vi "SECoP-addPropertyDouble.vi"(8 "error in (no error)":errorcluster, 9 "property value":dbl, 10 "property name":string, 11 "DLL path (in)":T1) -> (0 "error out":errorcluster, 3 "DLL path (out)":T1)   [LabVIEW 2023, in "SECoP.lvlib"]
doc: "Call <b>\"SECoP-addPropertyDouble.vi\"</b> to append a SECoP numeric property to the last SEC node, module, command or parameter. This is a convenience function like \"SECoP-addProperty.vi\" with a numeric double.\n\n<b>DLL path</b> input and output of cluster from \"SECoP-Initialize.vi\"\n<b>property name</b> name of property\n<b>property value</b> value of the property"
uses:
  SECoP.lvlib
  SECoP-libraries.ctl
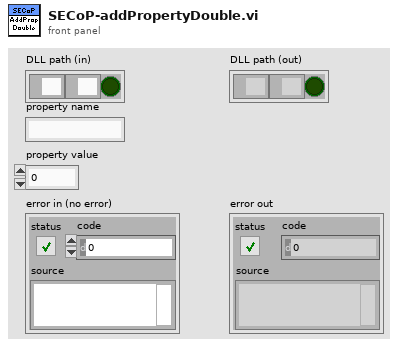
[diagram p1: front panel]
types:
  T1 = typedef "SECoP.lvlib/SECoP-libraries.ctl" = cluster{"serverDLL":path, "variantDLL":path, "cleanup_mode":bool}
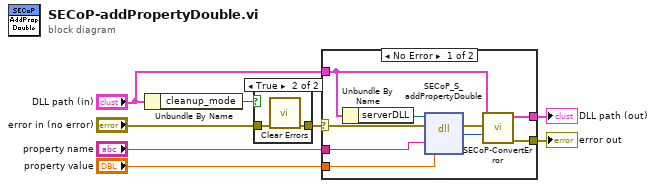
[diagram p0: block diagram]
diagram:
  n1 = Unbundle By Name("DLL path (in)") -> ("cleanup_mode"=w2:bool)
  n2 = case shown="True" w2 {
    tunnel: "error in (no error)" -> [w9 w11]
    tunnel: [w9 w10] -> w3
    frame False {
    }
    frame True {
      n3 = call <vilib>:"Clear Errors.vi"("error in (no error)"=w11) -> ("error out"=w10:errorcluster)  [unwired: 5 in, 1 out]
    }
  }
  n4 = case shown="No Error" w3 {
    selector: w3 -> [w18 w21]
    tunnel: "DLL path (in)" -> [w13 w22]
    tunnel: [w19 w22] -> w8
    tunnel: [w20 w21] -> w7
    tunnel: "property name" -> [w15 _]
    tunnel: "property value" -> [w14 _]
    frame No Error {
      n5 = Unbundle By Name(w13) -> ("serverDLL"=w12:path)
      n6 = dll-call lib="C:/Users/user/Desktop/x86_64/SECoP64.dll" fn="SECoP_S_addPropertyDouble"(path in=w12, error in=w18, "name"=w15, "value"=w14) -> (error out=w17:errorcluster, "return type"=w16:i32)  [unwired: 3 in, 1 out]
      n7 = call "SECoP-ConvertError.vi"("return code"=w16, "error in (no error)"=w17, "DLL path (in)"=w13) -> ("error out"=w20:errorcluster, "DLL path (out)"=w19:T1)  [unwired: 7 in]
    }
    frame Error {
    }
  }
  "DLL path (out)" <- w8
  "error out" <- w7
